vi "AuxConfig.vi"(8 "error in (no error)":errorcluster, 11 "Aux in":string[](array[string])) -> (0 "error out":errorcluster, 3 "Aux":string[](array[string]))   [LabVIEW 2014, in "MathLoop.lvlib"]
doc: "Configuración de los auxiliares."
uses:
  MathLoop.lvlib
  TypeDefs/ParsedExpression.ctl
  TypeDefs/typeMed.ctl
panel:
  in  "Cancel Aux":bool
  in  "Auxiliares":i32(listbox)
  in  "Add Aux":bool
  in  "Edit Aux":bool
  out "Nro Aux:":string="A1"
  in  "Delete Aux":bool
  in  "Stop Aux":bool
  in  "Formula:":string
  in  "Save Aux":bool
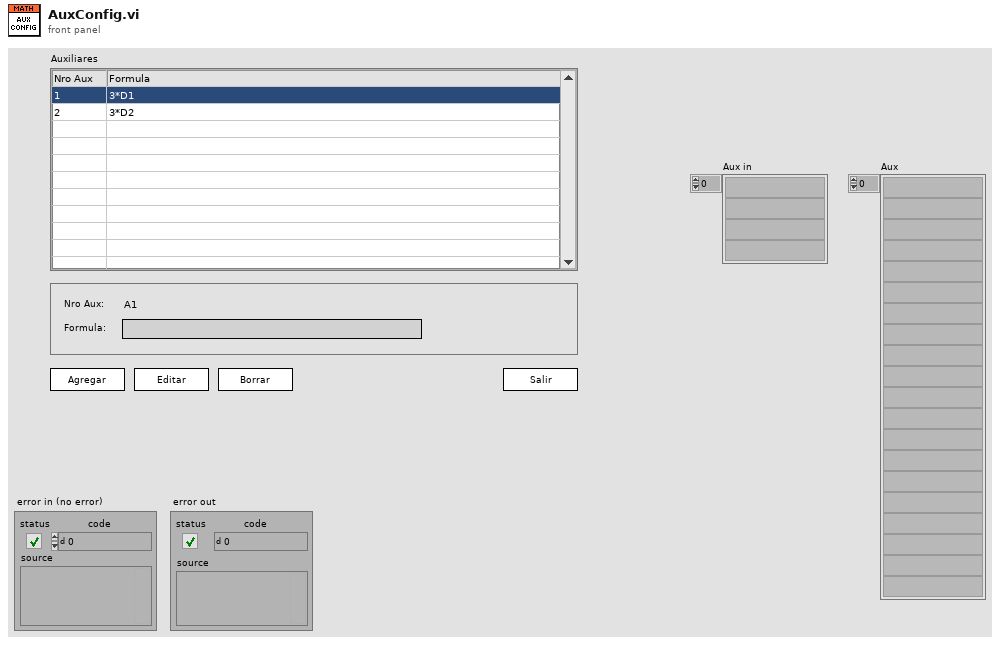
[diagram p1: front panel]
types:
  T1 = enum8{"Enabled", "Disabled", "Disabled and Grayed Out"}
  T2 = typedef "MathLoop.lvlib/ParsedExpression.ctl" = cluster{"RPN ":string[], "Constantes":sgl[], "Variables":string[], "Formula":string, "Tipo de Med":T3, "Med?":bool, "Descripción":string, "Nominal":sgl, "Tol Sup":sgl, "Pre TS":sgl, "Pre TI":sgl, "Tol Inf":sgl}
  T3 = typedef "MathLoop.lvlib/typeMed.ctl" = string
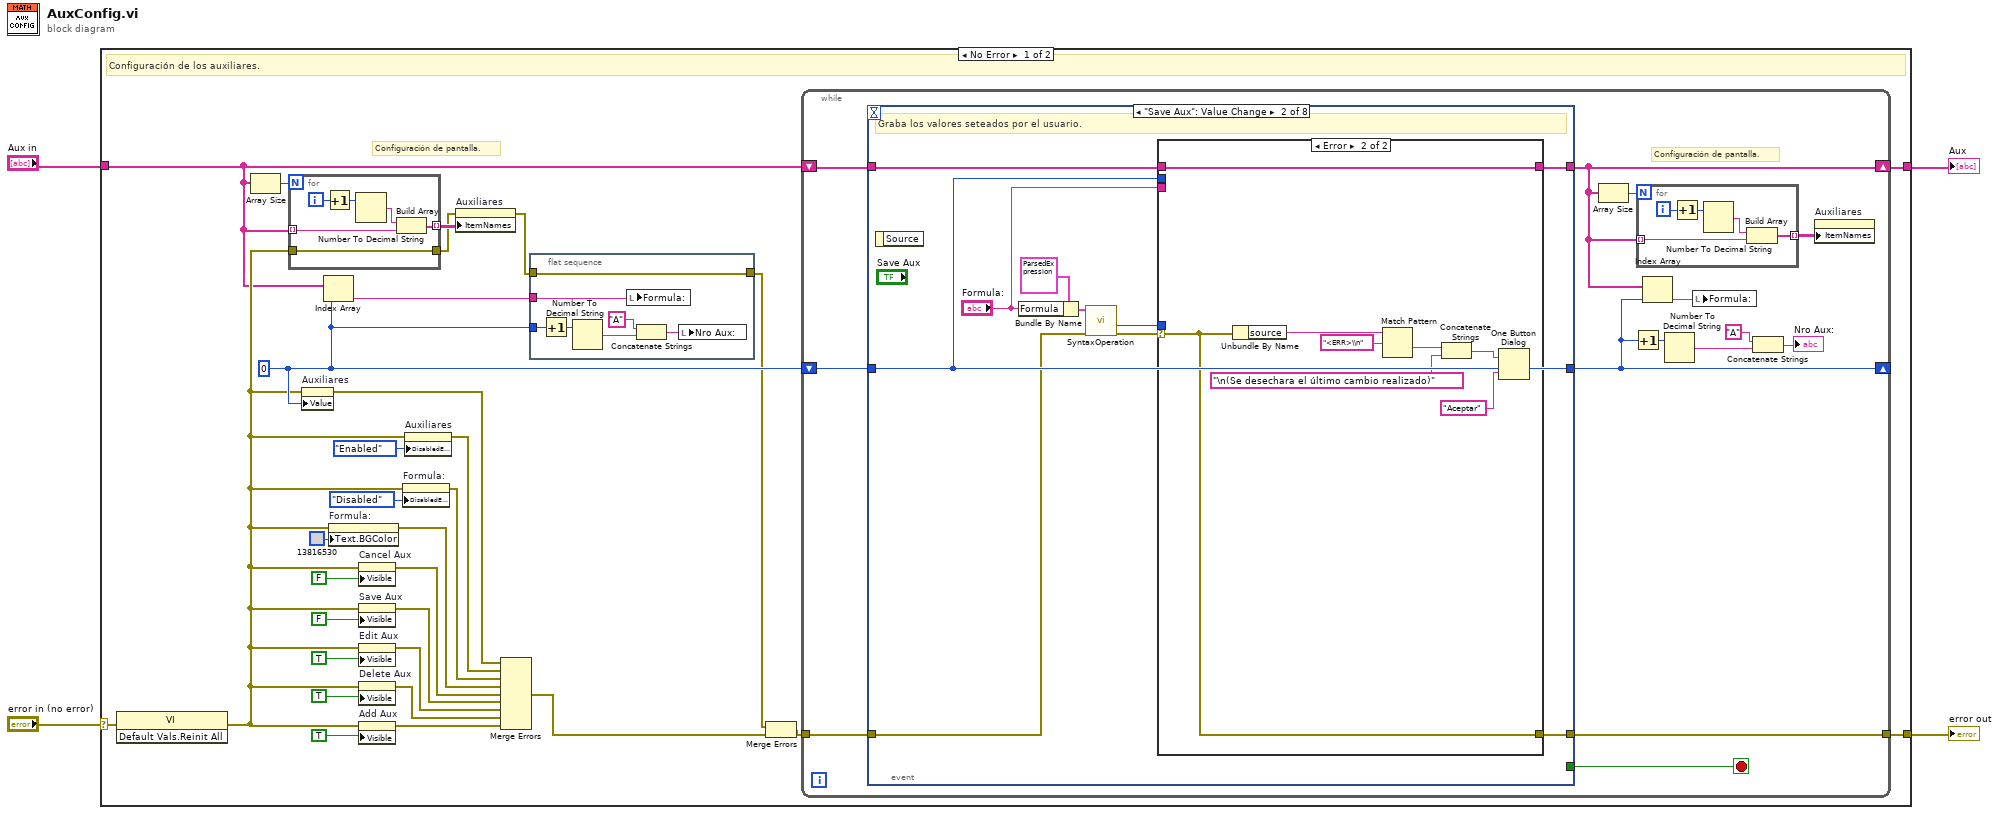
[diagram p0: block diagram]
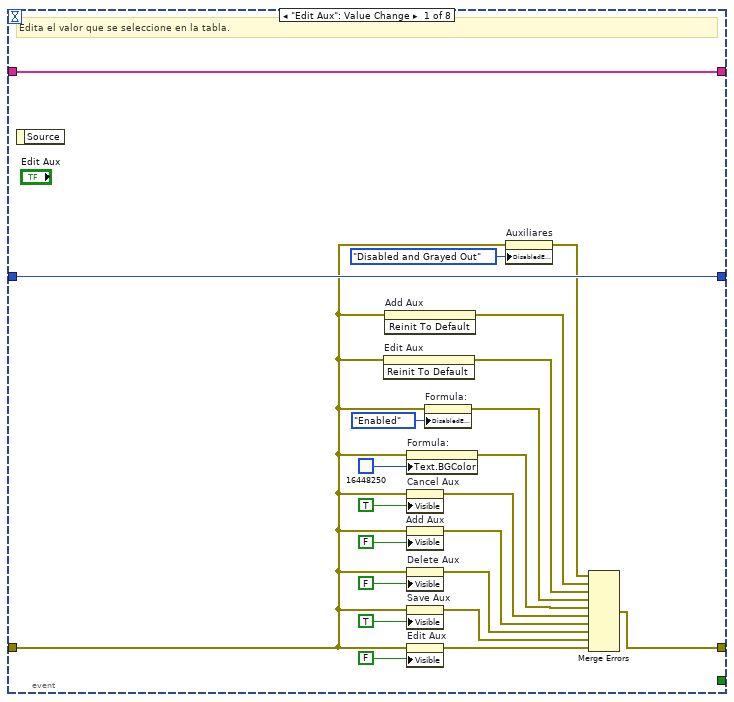
[diagram p2: hidden frame]
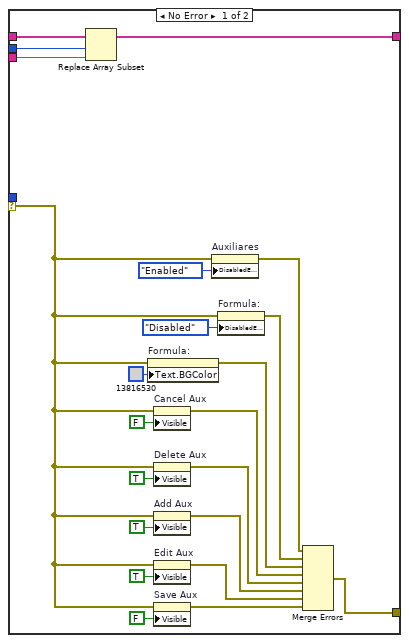
[diagram p3: hidden frame]
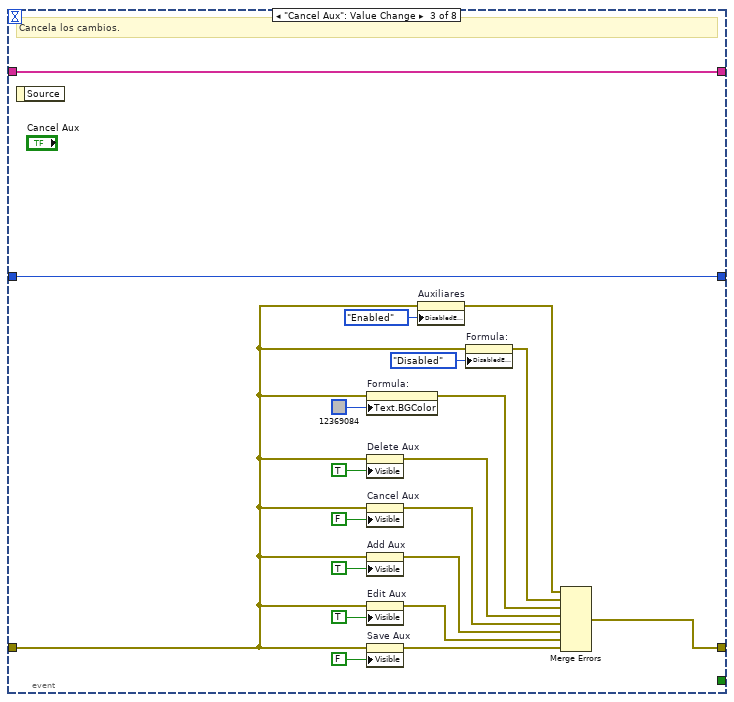
[diagram p4: hidden frame]
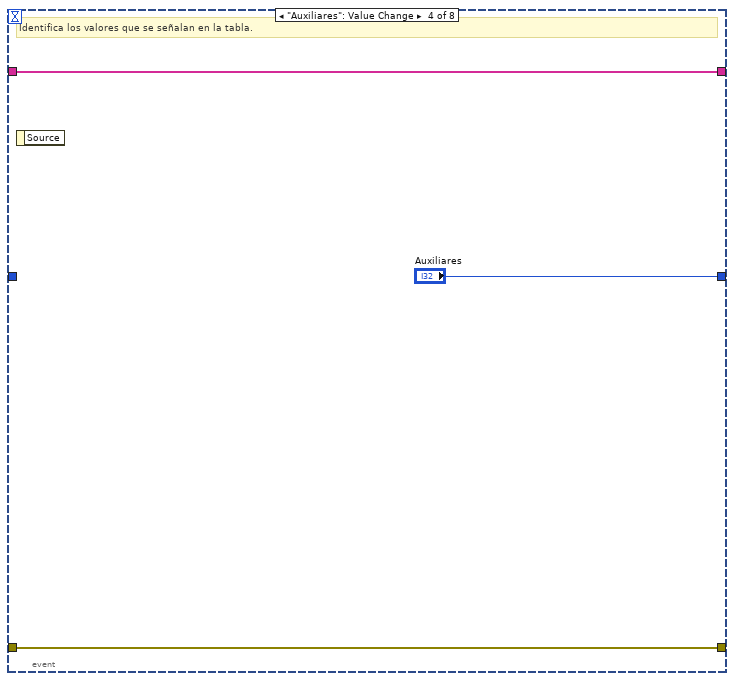
[diagram p5: hidden frame]
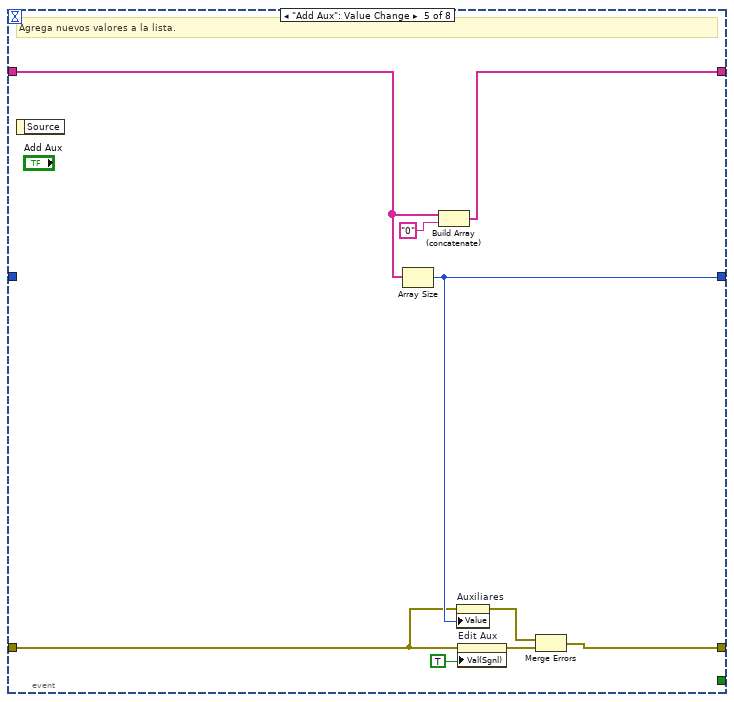
[diagram p6: hidden frame]
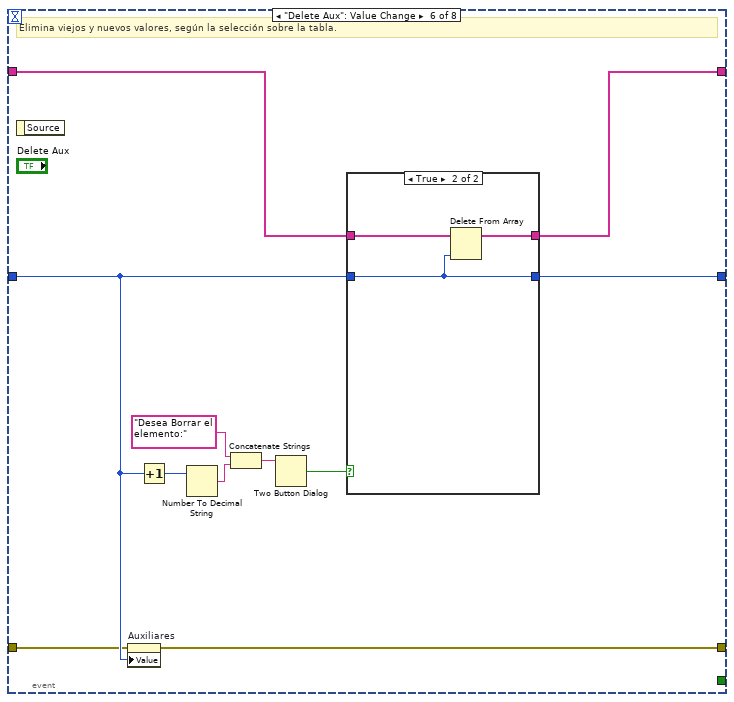
[diagram p7: hidden frame]
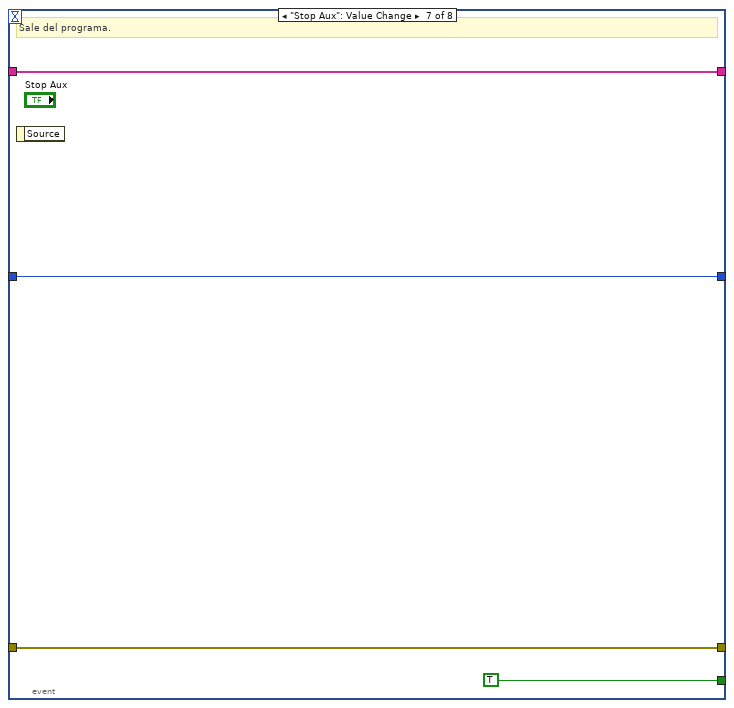
[diagram p9: hidden frame]
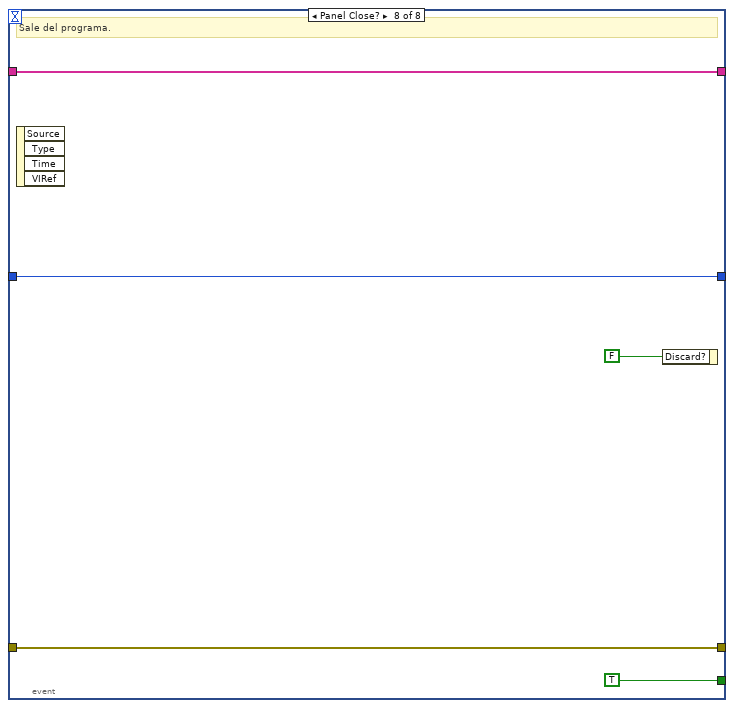
[diagram p10: hidden frame]
diagram:
  n1 = case shown="No Error" "error in (no error)" {
    selector: "error in (no error)" -> [w5 w188]
    tunnel: [w35 w188] -> w4
    tunnel: [w20 w187] -> w3
    tunnel: "Aux in" -> [w6 w187]
    frame No Error {
      w16 = 0 ("disabled index (col)")
      # "Configuración de pantalla."
      # "Configuración de los auxiliares."
      n2 = invoke class="VI" method="Default Vals.Reinit All"(error in=w5) -> (error out=w9:errorcluster)  [unwired: 2 in, 2 out]
      n3 = Array Size(array=w6) -> (size(s)=w29:i32)
      n4 = for {
        N: w29 -> [_]
        tunnel: w6 -> [w48] mode=indexing
        tunnel: [w46] -> w28 mode=indexing
        tunnel: w9 -> [w43]
        tunnel: [w43] -> w14
        i -> [w44]
        n5 = Increment(x=w44) -> (x+1=w45:i32)
        n6 = Number To Decimal String(number=w45) -> (decimal integer string=w47:string)  [unwired: 1 in]
        n7 = Build Array(w47, w48) -> (w46:string[])
      }
      n8 = property on="Auxiliares" class="MCListbox (strict)"(error in=w9, "Value"=w16) -> (error out=w7:errorcluster)  [unwired: 1 in, 1 out]
      n9 = Index Array(array=w6, index=w16) -> (element=w17:string)
      n10 = property on="Formula:" class="Str"(error in=w9, "Text.BGColor"=u32 13816530) -> (error out=w26:errorcluster)  [unwired: 1 in, 1 out]
      n11 = property on="Cancel Aux" class="Bool"(error in=w9, "Visible"=FALSE) -> (error out=w25:errorcluster)  [unwired: 1 in, 1 out]
      n12 = property on="Save Aux" class="Bool"(error in=w9, "Visible"=FALSE) -> (error out=w32:errorcluster)  [unwired: 1 in, 1 out]
      n13 = property on="Edit Aux" class="Bool (strict)"(error in=w9, "Visible"=TRUE) -> (error out=w31:errorcluster)  [unwired: 1 in, 1 out]
      n14 = property on="Delete Aux" class="Bool"(error in=w9, "Visible"=TRUE) -> (error out=w23:errorcluster)  [unwired: 1 in, 1 out]
      n15 = property on="Add Aux" class="Bool (strict)"(error in=w9, "Visible"=TRUE) -> (error out=w21:errorcluster)  [unwired: 1 in, 1 out]
      n16 = property on="Formula:" class="Str"(error in=w9, "DisabledEnum"=T1."Disabled" ("Disabled")) -> (error out=w18:errorcluster)  [unwired: 1 in, 1 out]
      n17 = property on="Auxiliares" class="MCListbox (strict)"(error in=w9, "DisabledEnum"=T1."Enabled" ("Disabled")) -> (error out=w8:errorcluster)  [unwired: 1 in, 1 out]
      n18 = property on="Auxiliares" class="MCListbox (strict)"(error in=w14, "ItemNames"=w28) -> (error out=w15:errorcluster)  [unwired: 1 in, 1 out]
      n19 = Merge Errors(w7, w8, w18, w26, w25, w32, w31, w23, w21) -> (w13:errorcluster)
      n20 = flat-sequence {
        tunnel: w17 -> [w39]
        tunnel: w16 -> [w37]
        tunnel: w15 -> [w36]
        tunnel: [w36] -> w11
        frame #0 {
          n21 = Increment(x=w37) -> (x+1=w41:i32)
          n22 = Number To Decimal String(number=w41) -> (decimal integer string=w42:string)  [unwired: 1 in]
          n23 = local write "Formula:"(w39) -> ()
          n24 = Concatenate Strings("A" ("string"), w42) -> (w38:string)
          n25 = local write "Nro Aux:"(w38) -> ()
        }
      }
      n26 = Merge Errors(w11, w13) -> (w12:errorcluster)
      n27 = while {
        shift-right: [w57] -> w20
        shift-left: w6 -> [w59]
        shift-right: [w56] -> _
        shift-left: w16 -> [w58]
        tunnel: w12 -> [w62]
        tunnel: [w61] -> w35
        stop <- w60 stop-if-true
        # "Configuración de pantalla."
        n28 = event shown="[1] \"Save Aux\": Value Change" {
          selector: _ -> [_ _ _ _ _ _ _ _]
          dyn-events: _ -> [_ _ _ _ _ _ _ _]
          timeout: _ -> [_ _ _ _ _ _ _ _]
          tunnel: w59 -> [w83 w98 w149 w152 w158 w170 w180 w186]
          tunnel: [w83 w97 w149 w152 w161 w169 w180 w186] -> w57
          tunnel: [w82 w99 w148 "Auxiliares" w157 w171 w179 w185] -> w56
          tunnel: w58 -> [w82 w99 w148 _ _ w164 w179 w185]
          tunnel: w62 -> [w69 w91 w130 w150 w154 w163 w181 w183]
          tunnel: [w84 w90 w140 w150 w153 w162 w181 w183] -> w61
          tunnel: [_ _ _ _ _ _ TRUE ("Stop Aux") TRUE ("Stop Aux")] -> w60
          event "Edit Aux": Value Change {
            # "Edita el valor que se seleccione en la tabla."
            n29 = event-data() -> ()  [unwired: 1 in, 1 out]
            n30 = invoke on="Edit Aux" class="Bool (strict)" method="Reinit To Default"(error in=w69) -> (error out=w72:errorcluster)  [unwired: 2 in, 2 out]
            n31 = invoke on="Add Aux" class="Bool (strict)" method="Reinit To Default"(error in=w69) -> (error out=w73:errorcluster)  [unwired: 2 in, 2 out]
            n32 = property on="Formula:" class="Str"(error in=w69, "Text.BGColor"=u32 16448250) -> (error out=w76:errorcluster)  [unwired: 1 in, 1 out]
            n33 = property on="Cancel Aux" class="Bool"(error in=w69, "Visible"=TRUE) -> (error out=w75:errorcluster)  [unwired: 1 in, 1 out]
            n34 = property on="Add Aux" class="Bool (strict)"(error in=w69, "Visible"=FALSE) -> (error out=w78:errorcluster)  [unwired: 1 in, 1 out]
            n35 = property on="Delete Aux" class="Bool"(error in=w69, "Visible"=FALSE) -> (error out=w80:errorcluster)  [unwired: 1 in, 1 out]
            n36 = property on="Save Aux" class="Bool"(error in=w69, "Visible"=TRUE) -> (error out=w85:errorcluster)  [unwired: 1 in, 1 out]
            n37 = property on="Edit Aux" class="Bool (strict)"(error in=w69, "Visible"=FALSE) -> (error out=w89:errorcluster)  [unwired: 1 in, 1 out]
            n38 = property on="Formula:" class="Str"(error in=w69, "DisabledEnum"=T1."Enabled" ("Disabled")) -> (error out=w71:errorcluster)  [unwired: 1 in, 1 out]
            n39 = property on="Auxiliares" class="MCListbox (strict)"(error in=w69, "DisabledEnum"=T1."Disabled and Grayed Out" ("Disabled")) -> (error out=w68:errorcluster)  [unwired: 1 in, 1 out]
            n40 = Merge Errors(w68, w73, w72, w71, w76, w75, w78, w80, w85, w89) -> (w84:errorcluster)
          }
          event "Save Aux": Value Change {
            # "Graba los valores seteados por el usuario."
            n41 = event-data() -> ()  [unwired: 1 in, 1 out]
            n42 = Bundle By Name(cluster=T2 {"RPN "=[], "Constantes"=[], "Variables"=[], "Formula"="", "Tipo de Med"="", "Med?"=FALSE, "Descripción"="", "Nominal"=0.0, "Tol Sup"=0.0, "Pre TS"=0.0, "Pre TI"=0.0, "Tol Inf"=0.0} ("Parsed Expression In"), "Formula"="Formula:") -> (w94:T2)
            n43 = call "SyntaxOperation.vi"("error in (no error)"=w91, "Parsed Expression In"=w94) -> ("error out"=w96:errorcluster, "Error Index Out"=w92:i32)  [unwired: 6 in, 2 out]
            n44 = case shown="Error" w96 {
              selector: w96 -> [w101 w122]
              tunnel: w99 -> [w121 _]
              tunnel: w98 -> [w120 w129]
              tunnel: [w119 w129] -> w97
              tunnel: "Formula:" -> [w118 _]
              tunnel: w92 -> [_ _]
              tunnel: [w105 w122] -> w90
              frame No Error {
                n45 = Replace Array Subset(array=w120, new element=w118, index=w121) -> (w119:string[])
                n46 = property on="Formula:" class="Str"(error in=w101, "Text.BGColor"=u32 13816530) -> (error out=w117:errorcluster)  [unwired: 1 in, 1 out]
                n47 = property on="Cancel Aux" class="Bool"(error in=w101, "Visible"=FALSE) -> (error out=w115:errorcluster)  [unwired: 1 in, 1 out]
                n48 = property on="Delete Aux" class="Bool"(error in=w101, "Visible"=TRUE) -> (error out=w116:errorcluster)  [unwired: 1 in, 1 out]
                n49 = property on="Add Aux" class="Bool (strict)"(error in=w101, "Visible"=TRUE) -> (error out=w112:errorcluster)  [unwired: 1 in, 1 out]
                n50 = property on="Edit Aux" class="Bool (strict)"(error in=w101, "Visible"=TRUE) -> (error out=w106:errorcluster)  [unwired: 1 in, 1 out]
                n51 = property on="Save Aux" class="Bool"(error in=w101, "Visible"=FALSE) -> (error out=w107:errorcluster)  [unwired: 1 in, 1 out]
                n52 = property on="Auxiliares" class="MCListbox (strict)"(error in=w101, "DisabledEnum"=T1."Enabled" ("Disabled")) -> (error out=w100:errorcluster)  [unwired: 1 in, 1 out]
                n53 = property on="Formula:" class="Str"(error in=w101, "DisabledEnum"=T1."Disabled" ("Disabled")) -> (error out=w103:errorcluster)  [unwired: 1 in, 1 out]
                n54 = Merge Errors(w100, w103, w117, w115, w116, w112, w106, w107) -> (w105:errorcluster)
              }
              frame Error {
                n55 = Unbundle By Name(w122) -> ("source"=w127:string)
                n56 = Match Pattern(string=w127, regular expression="<ERR>\\n") -> (after substring=w125:string)  [unwired: 1 in, 3 out]
                n57 = Concatenate Strings(w125, "\n(Se desechara el último cambio realizado)" ("button name (\"OK\")")) -> (w123:string)
                n58 = One Button Dialog(message=w123, button name ("OK")="Aceptar") -> ()  [unwired: 1 out]
              }
            }
          }
          event "Cancel Aux": Value Change {
            # "Cancela los cambios."
            n59 = event-data() -> ()  [unwired: 1 in, 1 out]
            n60 = property on="Formula:" class="Str"(error in=w130, "Text.BGColor"=u32 12369084) -> (error out=w137:errorcluster)  [unwired: 1 in, 1 out]
            n61 = property on="Delete Aux" class="Bool"(error in=w130, "Visible"=TRUE) -> (error out=w136:errorcluster)  [unwired: 1 in, 1 out]
            n62 = property on="Cancel Aux" class="Bool"(error in=w130, "Visible"=FALSE) -> (error out=w135:errorcluster)  [unwired: 1 in, 1 out]
            n63 = property on="Add Aux" class="Bool (strict)"(error in=w130, "Visible"=TRUE) -> (error out=w141:errorcluster)  [unwired: 1 in, 1 out]
            n64 = property on="Edit Aux" class="Bool (strict)"(error in=w130, "Visible"=TRUE) -> (error out=w147:errorcluster)  [unwired: 1 in, 1 out]
            n65 = property on="Save Aux" class="Bool"(error in=w130, "Visible"=FALSE) -> (error out=w146:errorcluster)  [unwired: 1 in, 1 out]
            n66 = property on="Auxiliares" class="MCListbox (strict)"(error in=w130, "DisabledEnum"=T1."Enabled" ("Disabled")) -> (error out=w131:errorcluster)  [unwired: 1 in, 1 out]
            n67 = property on="Formula:" class="Str"(error in=w130, "DisabledEnum"=T1."Disabled" ("Disabled")) -> (error out=w133:errorcluster)  [unwired: 1 in, 1 out]
            n68 = Merge Errors(w131, w133, w137, w136, w135, w141, w147, w146) -> (w140:errorcluster)
          }
          event "Auxiliares": Value Change {
            # "Identifica los valores que se señalan en la tabla."
            n69 = event-data() -> ()  [unwired: 1 in, 1 out]
          }
          event "Add Aux": Value Change {
            # "Agrega nuevos valores a la lista."
            n70 = event-data() -> ()  [unwired: 1 in, 1 out]
            n71 = Array Size(array=w158) -> (size(s)=w157:i32)
            n72 = Build Array (concatenate)(w158, "0") -> (w161:string[])
            n73 = property on="Auxiliares" class="MCListbox (strict)"(error in=w154, "Value"=w157) -> (error out=w156:errorcluster)  [unwired: 1 in, 1 out]
            n74 = property on="Edit Aux" class="Bool (strict)"(error in=w154, "Val(Sgnl)"=TRUE) -> (error out=w155:errorcluster)  [unwired: 1 in, 1 out]
            n75 = Merge Errors(w156, w155) -> (w153:errorcluster)
          }
          event "Delete Aux": Value Change {
            # "Elimina viejos y nuevos valores, según la selección sobre la tabla."
            n76 = event-data() -> ()  [unwired: 1 in, 1 out]
            n77 = property on="Auxiliares" class="MCListbox (strict)"(error in=w163, "Value"=w164) -> (error out=w162:errorcluster)  [unwired: 1 in, 1 out]
            n78 = Increment(x=w164) -> (x+1=w165:i32)
            n79 = Number To Decimal String(number=w165) -> (decimal integer string=w167:string)  [unwired: 1 in]
            n80 = Concatenate Strings("Desea Borrar el elemento:" ("message"), w167) -> (w166:string)
            n81 = Two Button Dialog(message=w166) -> (T button?=w172:bool)  [unwired: 2 in]
            n82 = case shown="True" w172 {
              tunnel: w170 -> [w173 w177]
              tunnel: [w174 w175] -> w171
              tunnel: w164 -> [w174 w175]
              tunnel: [w173 w176] -> w169
              frame False {
              }
              frame True {
                n83 = Delete From Array(array=w177, index=w175) -> (array with subset deleted=w176:string[])  [unwired: 1 in, 1 out]
              }
            }
          }
          event "Stop Aux": Value Change {
            # "Sale del programa."
            n84 = event-data() -> ()  [unwired: 1 in, 1 out]
          }
          event Panel Close? {
            # "Sale del programa."
            n85 = event-data() -> ()  [unwired: 1 in, 4 out]
            n86 = event-data("Discard?"=FALSE) -> ()  [unwired: 1 in, 1 out]
          }
        }
        n87 = Array Size(array=w57) -> (size(s)=w55:i32)
        n88 = Increment(x=w56) -> (x+1=w52:i32)
        n89 = for {
          N: w55 -> [_]
          tunnel: w57 -> [w67] mode=indexing
          tunnel: [w65] -> w54 mode=indexing
          i -> [w63]
          n90 = Increment(x=w63) -> (x+1=w64:i32)
          n91 = Number To Decimal String(number=w64) -> (decimal integer string=w66:string)  [unwired: 1 in]
          n92 = Build Array(w66, w67) -> (w65:string[])
        }
        n93 = Index Array(array=w57, index=w56) -> (element=w49:string)
        n94 = Number To Decimal String(number=w52) -> (decimal integer string=w53:string)  [unwired: 1 in]
        n95 = local write "Formula:"(w49) -> ()
        n96 = Concatenate Strings("A" ("string"), w53) -> (→"Nro Aux:":string)
        n97 = property on="Auxiliares" class="MCListbox (strict)"("ItemNames"=w54) -> ()  [unwired: 2 in, 2 out]
      }
    }
    frame Error {
    }
  }
  "error out" <- w4
  "Aux" <- w3
